vi "Calculate Angle and Amplitudes.vi"(10 "Current Phasors":csg[](array[numeric]), 11 "Voltage Phasors":csg[](array[numeric])) -> (0 "Reactive Power [MVAR]":dbl[](array[numeric]), 1 "Power [MW]":dbl[](array[numeric]), 2 "Current Amplitude [A]":dbl[](array[numeric]), 3 "Voltage Amplitude [kV]":dbl[](array[numeric]), 5 "Parameters":T1(array[ring])=[enum."Voltage", enum."Current", enum."Power", enum."Reactive Power", enum."Voltage Angle"])   [LabVIEW 2018, in "S3DK.lvlib" / "PMU Recorder Light.lvlib"]
uses:
  PMU Recorder Light.lvlib
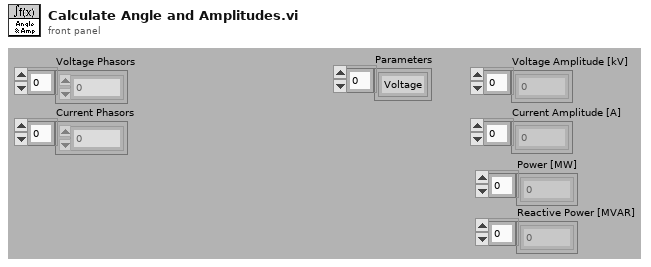
[diagram p1: front panel]
types:
  T1 = enum16{"Frequency", "Frequency Delta", "Voltage", "Voltage R", "Voltage S", "Voltage T", "Current", "Current R", "Current S", "Current T", "Voltage Amp", "Voltage Amp R", "Voltage Amp S", "Voltage Amp T", "Current Amp", "Current Amp R", "Current Amp S", "Current Amp T", "Voltage Angle", "Voltage Angle R", "Voltage Angle S", "Voltage Angle T", "Current Angle", "Current Angle R", "Current Angle S", "Current Angle T", "Angle Difference", "Power", "Reactive Power", "Unknown"}[]
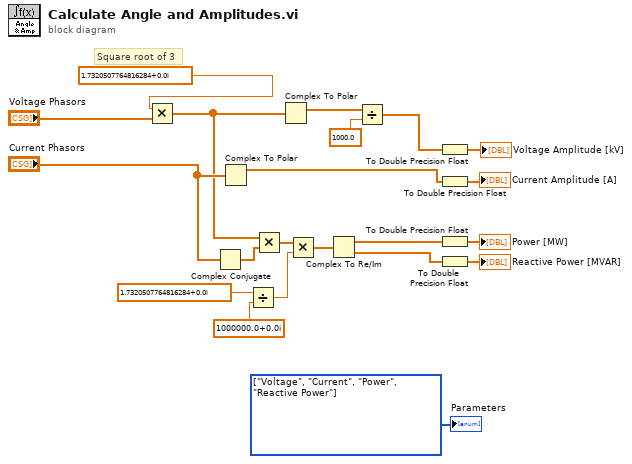
[diagram p0: block diagram]
diagram:
  w11 = T1 [enum."Voltage", enum."Current", enum."Power", enum."Reactive Power"] items=["Frequency", "Frequency Delta", "Voltage", "Voltage R", "Voltage S", "Voltage T", "Current", "Current R", "Current S", "Current T", "Voltage Amp", "Voltage Amp R", "Voltage Amp S", "Voltage Amp T", "Current Amp", "Current Amp R", "Current Amp S", "Current Amp T", "Voltage Angle", "Voltage Angle R", "Voltage Angle S", "Voltage Angle T", "Current Angle", "Current Angle R", "Current Angle S", "Current Angle T", "Angle Difference", "Power", "Reactive Power", "Unknown"]
  # "Square root of 3"
  n1 = Multiply(x=csg 1.7320508+0.0i ("Numeric 2"), y="Voltage Phasors") -> (x*y=w1:csg[])
  n2 = Complex Conjugate(1:"Current Phasors") -> (0:w16:csg[])
  n3 = Complex To Polar(r * e^(i*theta)="Current Phasors") -> (r=w7:sgl[])  [unwired: 1 out]
  n4 = Divide(x=csg 1.7320508+0.0i ("Numeric 2"), y=csg 1000000.0+0.0i) -> (x/y=w20:csg)
  n5 = Multiply(x=w1, y=w16) -> (x*y=w18:csg[])
  n6 = Complex To Polar(r * e^(i*theta)=w1) -> (r=w15:sgl[])  [unwired: 1 out]
  n7 = Multiply(x=w18, y=w20) -> (x*y=w21:csg[])
  n8 = Complex To Re/Im(x + iy=w21) -> (x=w6:sgl[], y=w5:sgl[])
  n9 = Divide(x=w15, y=sgl 1000.0) -> (x/y=w10:sgl[])
  n10 = To Double Precision Float(number=w10) -> (double precision float=→"Voltage Amplitude [kV]":dbl[])
  n11 = To Double Precision Float(number=w7) -> (double precision float=→"Current Amplitude [A]":dbl[])
  n12 = To Double Precision Float(number=w6) -> (double precision float=→"Power [MW]":dbl[])
  n13 = To Double Precision Float(number=w5) -> (double precision float=→"Reactive Power [MVAR]":dbl[])
  "Parameters" <- w11
